vi "Get Display Queue.vi"(8 "error in (no error)":errorcluster, 10 "create if not found? (T)":bool) -> (0 "error out":errorcluster, 3 "Queue out":refnum<queue>)   [LabVIEW 2018, in "Assert API Components.lvlib" / "Assert Display.lvlib"]
uses:
  Assert Display.lvlib
  Assert Display/Assert Display.lvclass
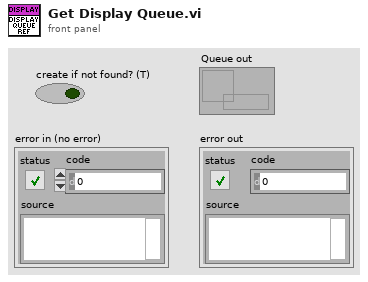
[diagram p1: front panel]
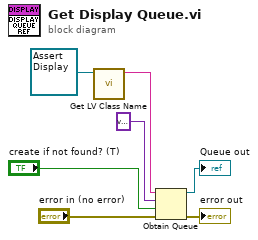
[diagram p0: block diagram]
diagram:
  n1 = call <vilib>:"Get LV Class Name.vi"("object"=refnum<class "Assert Display.lvclass"> refnum ("Assert API Components.lvlib:Assert Display.lvlib:Assert Display.lvclass")) -> ("class name"=w2:string)  [unwired: 9 in, 1 out]
  n2 = Obtain Queue(name (unnamed)=w2, element data type=variant, create if not found? (T)="create if not found? (T)", error in (no error)="error in (no error)") -> (queue out=→"Queue out":refnum<queue>, error out=→"error out":errorcluster)  [unwired: 1 in, 1 out]
